vi "Read Device Identification.vi"(8 "error in (no error)":errorcluster, 9 "object ID":u8, 10 "read device ID code":T1(ring), 11 "Modbus instance in":refnum<class "Modbus API.lvclass">) -> (0 "error out":errorcluster, 2 "objects":cluster{"object ID":u8, "value":string}[](array[cluster]) {"object ID" format="%x"}, 3 "Modbus instance out":refnum<class "Modbus API.lvclass">)   [LabVIEW 2020, in "SubVIs.lvlib" / "Modbus API.lvclass"]
doc: "Reads Modbus object information stored on the device. This can include basic information, like manufacturer, additional standard items, or model-specific extended items. This function may take a large amount of time to execute, as it requires the transfer of a large quantity of binary data. Even on TCP/IP, this function is limited by the maximum defined size of a Modbus protocol data unit."
uses:
  <vilib>/Modbus/subvis/Modbus API/Modbus API.lvclass
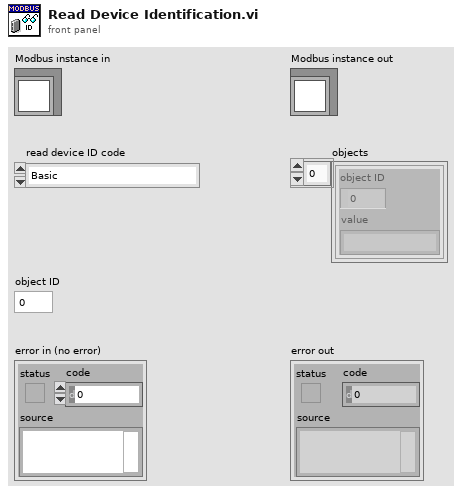
[diagram p1: front panel]
types:
  T1 = enum8{"Basic", "Regular", "Extended", "Specific"}
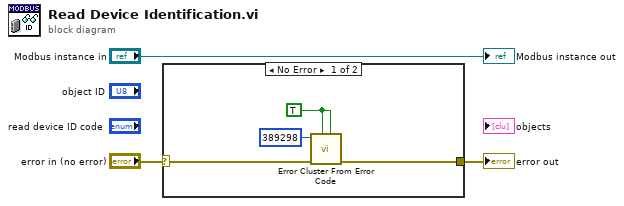
[diagram p0: block diagram]
diagram:
  n1 = case shown="No Error" "error in (no error)" {
    selector: "error in (no error)" -> [w6 w8]
    tunnel: [w7 w8] -> w1
    frame No Error {
      w4 = TRUE ("show call chain? (False)")
      n2 = call <vilib>:"Error Cluster From Error Code.vi"("is warning? (False)"=w4, "show call chain? (False)"=w4, "error in (no error)"=w6, "error code (0)"=389298) -> ("error out"=w7:errorcluster)  [unwired: 5 in]
    }
    frame Error {
    }
  }
  "error out" <- w1
  "Modbus instance out" <- "Modbus instance in"
